vi "Clear_Data_Tomography_v1.vi"(0 "ZI Data 0/3":T1[](array[typedef]), 2 "Fixed Number Of Points":bool, 3 "Check Phase Mismatch":bool, 5 "Time Of Collected Data (ms)":dbl=500.0, 7 "Fixed Number Of Points":u16 min=1, 9 "Crosstalk Tolerance":dbl=0.1, 11 "error in":errorcluster) -> (4 "Cutted Data":T2, 6 "Cutted Data 3":T2, 12 "Trig Out Found(?)":bool, 13 "Enough Points (?)":bool, 14 "Possible Mismatch In Phase (?)":bool, 15 "error out":errorcluster)   [LabVIEW 2021]
uses:
  Ver_1/Cutted_Data.ctl
  Ver_1/ZI_Data.ctl
  <vilib>/Utility/error.llb/Error Cluster From Error Code.vi
  <vilib>/ErrorRing/Error Ring.xnode
  <vilib>/Analysis/NI_AALBase.lvlib
panel:
  out "first subarray":dbl[](array[numeric])
  out "subarray":dbl[](array[numeric])
  out "standard deviation 2":dbl format="%e"
  out "x*y 2":dbl
  out "x*y":dbl
  out "standard deviation":dbl format="%e"
  out "Probe Stop (s)":dbl
  out "Probe Stop (i)":i32
  out "Probe Mag Field Start (s)":dbl
  out "Probe Mag Field Start (i)":i32
  # "cutting data on demod 0 AuxIn0"
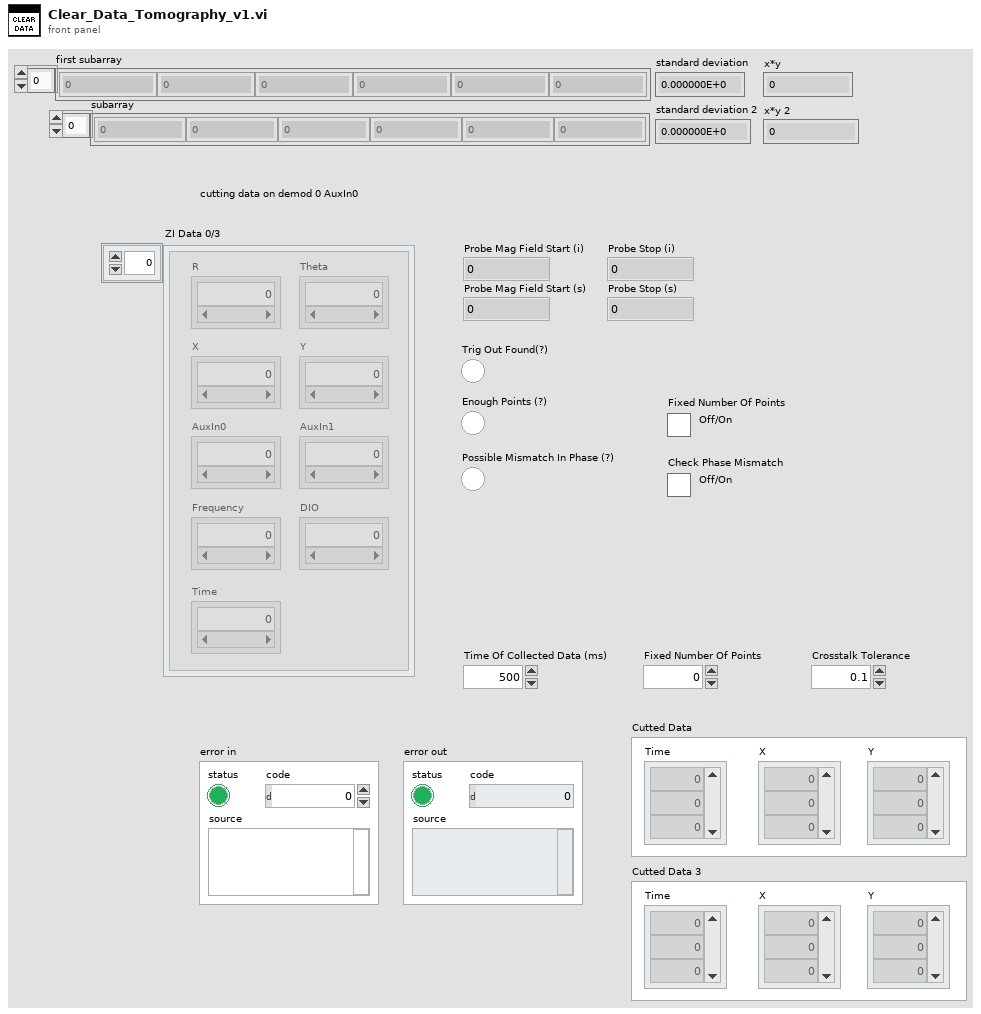
[diagram p1: front panel]
types:
  T1 = typedef "ZI_Data.ctl" = cluster{"R":dbl[], "Theta":dbl[], "X":dbl[], "Y":dbl[], "AuxIn0":dbl[], "AuxIn1":dbl[], "Frequency":dbl[], "DIO":dbl[], "Time":dbl[]}
  T2 = typedef "Cutted_Data.ctl" = cluster{"X":dbl[], "Y":dbl[], "Time":dbl[]}
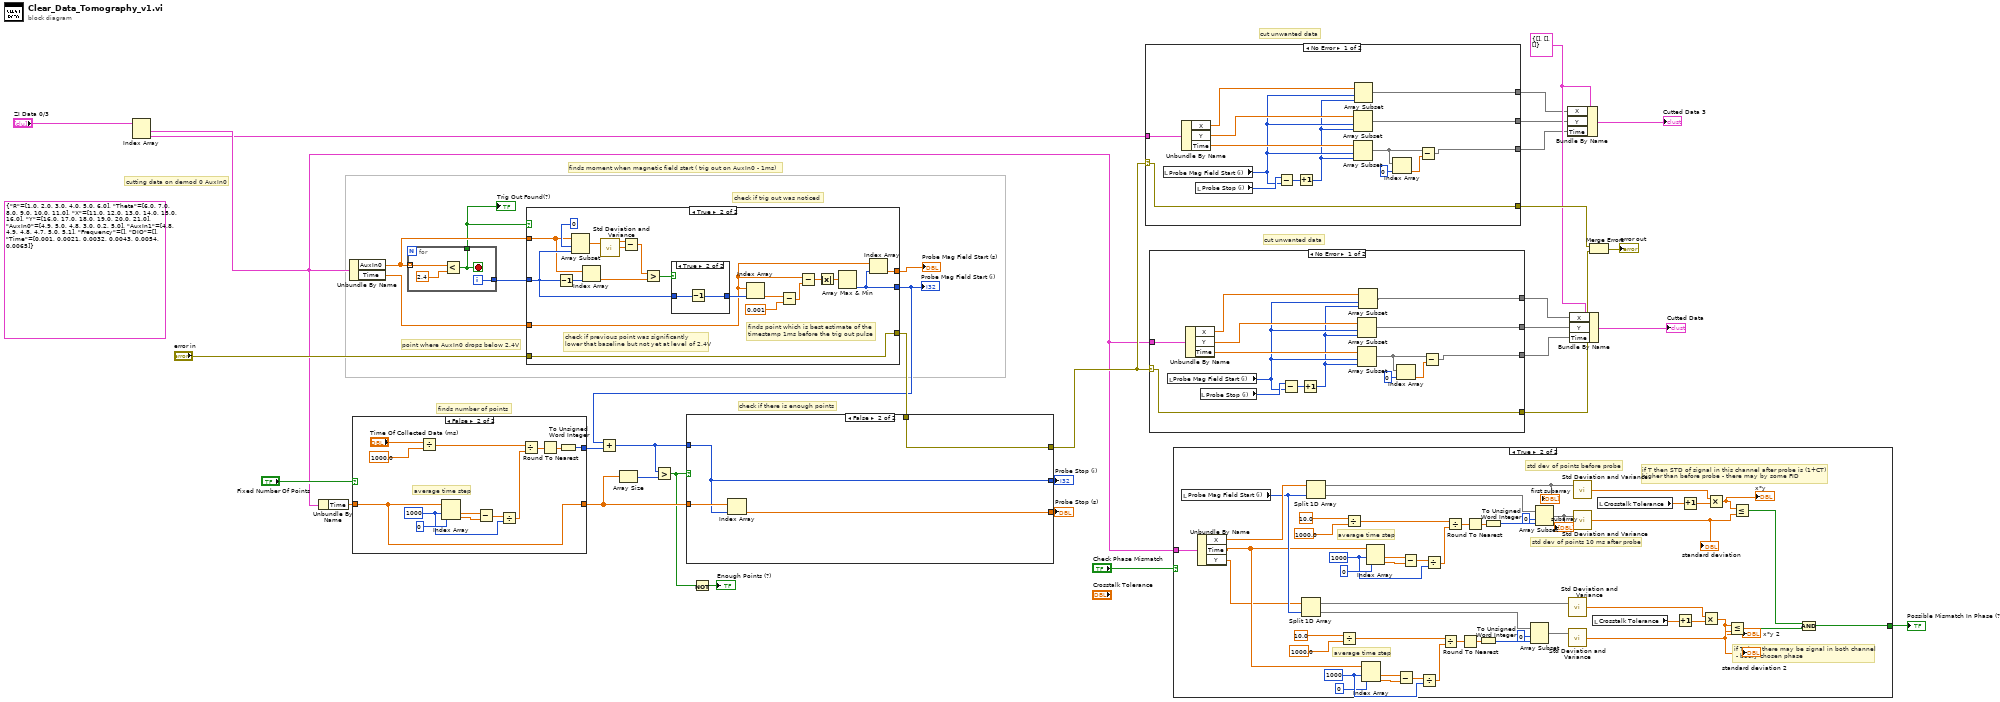
[diagram p0: block diagram]
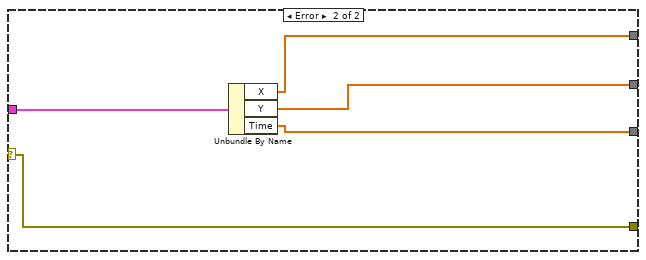
[diagram p2: hidden frame]
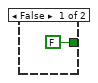
[diagram p3: hidden frame]
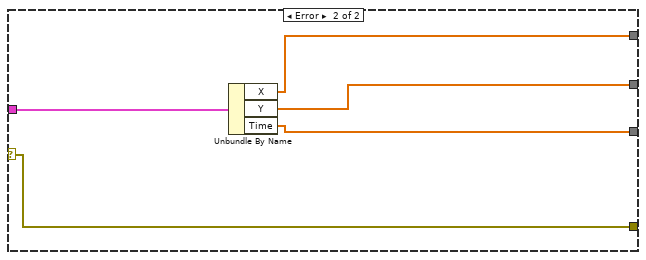
[diagram p4: hidden frame]
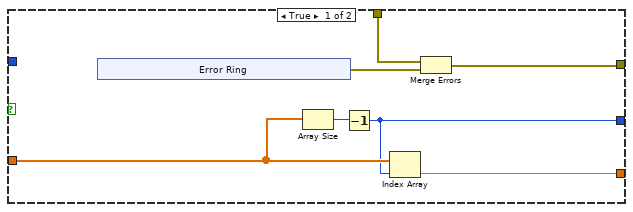
[diagram p5: hidden frame]
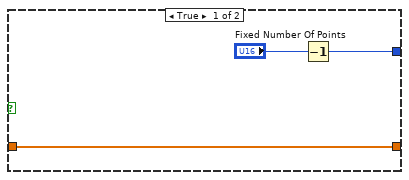
[diagram p6: hidden frame]
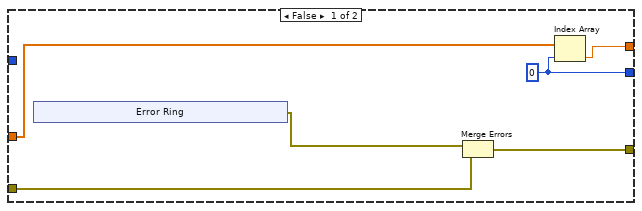
[diagram p7: hidden frame]
diagram:
  w13 = T2 {"X"=[], "Y"=[], "Time"=[]} ("Cutted Data 2")
  (unwired) T1 {"R"=[1.0, 2.0, 3.0, 4.0, 5.0, 6.0], "Theta"=[6.0, 7.0, 8.0, 9.0, 10.0, 11.0], "X"=[11.0, 12.0, 13.0, 14.0, 15.0, 16.0], "Y"=[16.0, 17.0, 18.0, 19.0, 20.0, 21.0], "AuxIn0"=[4.9, 5.0, 4.8, 3.0, 0.2, 5.0], "AuxIn1"=[4.8, 4.9, 4.8, 4.7, 5.0, 5.1], "Frequency"=[], "DIO"=[], "Time"=[0.001, 0.0021, 0.0032, 0.0043, 0.0054, 0.0065]} ("ZI Data")
  # "cut unwanted data"
  # "cutting data on demod 0 AuxIn0"
  # "cut unwanted data"
  # "check if there is enough points"
  # "finds number of points"
  # "check if trig out was noticed"
  # "point where AuxIn0 drops below 2.4V"
  # "finds moment when magnetic field start ( trig out on AuxIn0 - 1ms)"
  n1 = Index Array(array="ZI Data 0/3") -> (element #1=w2:T1, element #2=w1:T1)  [unwired: 2 in]
  n2 = Unbundle By Name(w2) -> ("Time"=w28:dbl[])
  n3 = Unbundle By Name(w2) -> ("AuxIn0"=w35:dbl[], "Time"=w34:dbl[])
  n4 = case shown="False" "Fixed Number Of Points" {
    tunnel: [w37 w41] -> w29
    tunnel: w28 -> [w39 w40]
    tunnel: [w39 w40] -> w26
    frame True {
      n5 = Decrement(x="Fixed Number Of Points") -> (x-1=w37:u16)
    }
    frame False {
      w46 = 1000 ("index")
      # "average time step"
      n6 = Divide(x="Time Of Collected Data (ms)", y=1000.0) -> (x/y=w45:dbl)
      n7 = Index Array(array=w40, index #1=w46, index #2=0 ("index")) -> (element #1=w49:dbl, element #2=w48:dbl)
      n8 = Subtract(x=w49, y=w48) -> (x-y=w47:dbl)
      n9 = Divide(x=w47, y=w46) -> (x/y=w44:dbl)
      n10 = Divide(x=w45, y=w44) -> (x/y=w43:dbl)
      n11 = Round To Nearest(number=w43) -> (nearest integer value=w42:dbl)
      n12 = To Unsigned Word Integer(number=w42) -> (unsigned 16bit integer=w41:u16)
    }
  }
  n13 = for {
    tunnel: w35 -> [w56] mode=indexing
    tunnel: [w54] -> w36
    tunnel: [w53] -> w31
    i -> [w54]
    stop <- w53 stop-if-true
    n14 = Less?(x=w56, y=2.4) -> (x < y?=w53:bool)
  }
  "Trig Out Found(?)" <- w31
  n15 = case shown="True" w31 {
    tunnel: w36 -> [_ w79]
    tunnel: w35 -> [_ w77]
    tunnel: [w58 w73] -> w4
    tunnel: w34 -> [w59 w72]
    tunnel: [w57 w71] -> w33
    tunnel: "error in" -> [w62 w68]
    tunnel: [w60 w68] -> w22
    frame False {
      w58 = 0
      n16 = xnode "Error Ring"() -> ("error out"=w61:errorcluster)
      n17 = Merge Errors(w61, w62) -> (w60:errorcluster)
      n18 = Index Array(array=w59, index=w58) -> (element=w57:dbl)
    }
    frame True {
      # "finds point which is best estimate of the\ntimestamp 1ms before the trig out pulse"
      # "check if previous point was significantly\nlower that baseline but not yet at level of 2.4V"
      n19 = Decrement(x=w79) -> (x-1=w85:i32)
      n20 = Array Subset(array=w77, index=0, length=w79) -> (w86:dbl[])
      n21 = Index Array(array=w77, index=w85) -> (element=w81:dbl)
      n22 = call <vilib>:"Std Deviation and Variance.vi"("X"=w86) -> ("mean"=w84:dbl, "standard deviation"=w83:dbl)  [unwired: 1 in, 1 out]
      n23 = Subtract(x=w84, y=w83) -> (x-y=w82:dbl)
      n24 = Greater?(x=w82, y=w81) -> (0:w80:bool)
      n25 = case shown="True" w80 {
        tunnel: w79 -> [w88 w90]
        tunnel: [w88 w89] -> w78
        frame False {
        }
        frame True {
          n26 = Decrement(x=w90) -> (x-1=w89:i32)
        }
      }
      n27 = Index Array(array=w72, index=w78) -> (element=w76:dbl)
      n28 = Subtract(x=w76, y=0.001) -> (x-y=w74:dbl)
      n29 = Subtract(x=w72, y=w74) -> (x-y=w69:dbl[])
      n30 = Absolute Value(x=w69) -> (abs(x)=w70:dbl[])
      n31 = Array Max & Min(array=w70) -> (min index (indices)=w73:i32)  [unwired: 3 out]
      n32 = Index Array(array=w72, index=w73) -> (element=w71:dbl)
    }
  }
  "Probe Mag Field Start (i)" <- w4
  "Probe Mag Field Start (s)" <- w33
  n33 = Add(x=w4, y=w29) -> (x+y=w25:i32)
  n34 = Array Size(array=w26) -> (size(s)=w27:i32)
  n35 = Greater?(x=w25, y=w27) -> (0:w20:bool)
  n36 = case shown="False" w20 {
    tunnel: w26 -> [w93 w106]
    tunnel: w25 -> [_ w104]
    tunnel: [w92 w105] -> w24
    tunnel: [w91 w104] -> w23
    tunnel: w22 -> [w95 w103]
    tunnel: [w97 w103] -> w14
    frame True {
      n37 = xnode "Error Ring"() -> ("error out"=w96:errorcluster)
      n38 = Array Size(array=w93) -> (size(s)=w94:i32)
      n39 = Decrement(x=w94) -> (x-1=w91:i32)
      n40 = Index Array(array=w93, index=w91) -> (element=w92:dbl)
      n41 = Merge Errors(w95, w96) -> (w97:errorcluster)
    }
    frame False {
      n42 = Index Array(array=w106, index=w104) -> (element=w105:dbl)
    }
  }
  "Probe Stop (i)" <- w23
  "Probe Stop (s)" <- w24
  n43 = Not(x=w20) -> (.not. x?=→"Enough Points (?)":bool)
  n44 = case shown="No Error" w14 {
    selector: w14 -> [w111 w122]
    tunnel: w1 -> [w121 w126]
    tunnel: [w113 w125] -> w12
    tunnel: [w112 w124] -> w11
    tunnel: [w107 w123] -> w10
    tunnel: [w111 w122] -> w17
    frame No Error {
      n45 = local read "Probe Mag Field Start (i)"() -> (w115:i32)
      n46 = Unbundle By Name(w121) -> ("X"=w117:dbl[], "Y"=w116:dbl[], "Time"=w119:dbl[])
      n47 = local read "Probe Stop (i)"() -> (w120:i32)
      n48 = Subtract(x=w120, y=w115) -> (x-y=w118:i32)
      n49 = Increment(x=w118) -> (x+1=w114:i32)
      n50 = Array Subset(array=w116, index=w115, length=w114) -> (w112:dbl[])
      n51 = Array Subset(array=w119, index=w115, length=w114) -> (w110:dbl[])
      n52 = Array Subset(array=w117, index=w115, length=w114) -> (w113:dbl[])
      n53 = Index Array(array=w110, index=0) -> (element=w109:dbl)
      n54 = Subtract(x=w110, y=w109) -> (x-y=w107:dbl[])
    }
    frame Error {
      n55 = Unbundle By Name(w126) -> ("X"=w125:dbl[], "Y"=w124:dbl[], "Time"=w123:dbl[])
    }
  }
  n56 = case shown="No Error" w14 {
    selector: w14 -> [w131 w142]
    tunnel: w2 -> [w141 w146]
    tunnel: [w133 w145] -> w7
    tunnel: [w132 w144] -> w8
    tunnel: [w127 w143] -> w6
    tunnel: [w131 w142] -> w16
    frame No Error {
      n57 = local read "Probe Mag Field Start (i)"() -> (w135:i32)
      n58 = Unbundle By Name(w141) -> ("X"=w137:dbl[], "Y"=w136:dbl[], "Time"=w139:dbl[])
      n59 = local read "Probe Stop (i)"() -> (w140:i32)
      n60 = Subtract(x=w140, y=w135) -> (x-y=w138:i32)
      n61 = Increment(x=w138) -> (x+1=w134:i32)
      n62 = Array Subset(array=w136, index=w135, length=w134) -> (w132:dbl[])
      n63 = Array Subset(array=w139, index=w135, length=w134) -> (w130:dbl[])
      n64 = Array Subset(array=w137, index=w135, length=w134) -> (w133:dbl[])
      n65 = Index Array(array=w130, index=0) -> (element=w129:dbl)
      n66 = Subtract(x=w130, y=w129) -> (x-y=w127:dbl[])
    }
    frame Error {
      n67 = Unbundle By Name(w146) -> ("X"=w145:dbl[], "Y"=w144:dbl[], "Time"=w143:dbl[])
    }
  }
  n68 = case shown="True" "Check Phase Mismatch" {
    tunnel: w2 -> [_ w197]
    tunnel: [FALSE w152] -> w19
    frame False {
    }
    frame True {
      w163 = 1000 ("index")
      w191 = 1000 ("index")
      # "if T then there may be signal in both channel\n - badly chosen phase"
      # "average time step"
      # "if T then STD of signal in this channel after probe is (1+CT) \nhigher than before probe - there may by some FID"
      # "std dev of points 10 ms after probe"
      # "std dev of points before probe"
      # "average time step"
      n69 = local read "Probe Mag Field Start (i)"() -> (w157:i32)
      n70 = Unbundle By Name(w197) -> ("X"=w185:dbl[], "Time"=w156:dbl[], "Y"=w155:dbl[])
      n71 = Split 1D Array(array=w155, index=w157) -> (first subarray=w169:dbl[], second subarray=w171:dbl[])
      n72 = Split 1D Array(array=w185, index=w157) -> (first subarray=w184:dbl[], second subarray=w182:dbl[])
      "first subarray" <- w184
      n73 = Divide(x=10.0, y=1000.0) -> (x/y=w164:dbl)
      n74 = Divide(x=10.0, y=1000.0) -> (x/y=w190:dbl)
      n75 = Index Array(array=w156, index #1=w163, index #2=0 ("index")) -> (element #1=w160:dbl, element #2=w161:dbl)
      n76 = Index Array(array=w156, index #1=w191, index #2=0 ("index")) -> (element #1=w194:dbl, element #2=w193:dbl)
      n77 = Subtract(x=w160, y=w161) -> (x-y=w162:dbl)
      n78 = Subtract(x=w194, y=w193) -> (x-y=w192:dbl)
      n79 = Divide(x=w162, y=w163) -> (x/y=w165:dbl)
      n80 = Divide(x=w192, y=w191) -> (x/y=w189:dbl)
      n81 = Divide(x=w164, y=w165) -> (x/y=w166:dbl)
      n82 = Divide(x=w190, y=w189) -> (x/y=w188:dbl)
      n83 = Round To Nearest(number=w166) -> (nearest integer value=w167:dbl)
      n84 = Round To Nearest(number=w188) -> (nearest integer value=w187:dbl)
      n85 = To Unsigned Word Integer(number=w167) -> (unsigned 16bit integer=w170:u16)
      n86 = To Unsigned Word Integer(number=w187) -> (unsigned 16bit integer=w183:u16)
      n87 = Array Subset(array=w171, index=0, length=w170) -> (w172:dbl[])
      n88 = Array Subset(array=w182, index=0, length=w183) -> (w181:dbl[])
      "subarray" <- w181
      n89 = call <vilib>:"Std Deviation and Variance.vi"("X"=w169) -> ("standard deviation"=w175:dbl)  [unwired: 1 in, 2 out]
      n90 = call <vilib>:"Std Deviation and Variance.vi"("X"=w172) -> ("standard deviation"=w177:dbl)  [unwired: 1 in, 2 out]
      "standard deviation 2" <- w177
      n91 = call <vilib>:"Std Deviation and Variance.vi"("X"=w184) -> ("standard deviation"=w149:dbl)  [unwired: 1 in, 2 out]
      n92 = call <vilib>:"Std Deviation and Variance.vi"("X"=w181) -> ("standard deviation"=w178:dbl)  [unwired: 1 in, 2 out]
      "standard deviation" <- w178
      n93 = local read "Crosstalk Tolerance"() -> (w173:dbl)
      n94 = local read "Crosstalk Tolerance"() -> (w180:dbl)
      n95 = Increment(x=w173) -> (x+1=w174:dbl)
      n96 = Increment(x=w180) -> (x+1=w179:dbl)
      n97 = Multiply(x=w175, y=w174) -> (x*y=w176:dbl)
      "x*y 2" <- w176
      n98 = Multiply(x=w149, y=w179) -> (x*y=w148:dbl)
      "x*y" <- w148
      n99 = Less Or Equal?(x=w176, y=w177) -> (x <= y?=w153:bool)
      n100 = Less Or Equal?(x=w148, y=w178) -> (x <= y?=w154:bool)
      n101 = And(x=w154, y=w153) -> (x .and. y?=w152:bool)
    }
  }
  "Possible Mismatch In Phase (?)" <- w19
  n102 = Bundle By Name(cluster=w13, "X"=w12, "Y"=w11, "Time"=w10) -> (→"Cutted Data 3":T2)
  n103 = Bundle By Name(cluster=w13, "X"=w7, "Y"=w8, "Time"=w6) -> (→"Cutted Data":T2)
  n104 = Merge Errors(w17, w16) -> (→"error out":errorcluster)
